vi "Read U64.vi"(8 "error in":errorcluster, 10 "register name":string, 11 "session in":u32) -> (0 "error out":errorcluster, 2 "value out":u64, 3 "session out":u32)   [LabVIEW 2018, in "Scalar IO Operations.lvlib"]
uses:
  Scalar IO Operations.lvlib
  NiFpga.dll
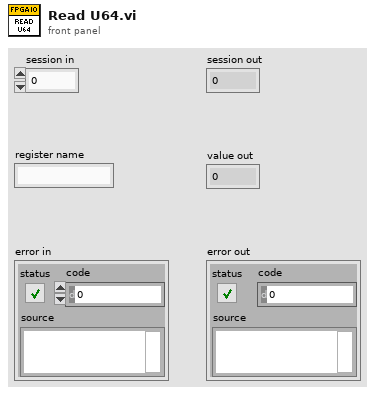
[diagram p1: front panel]
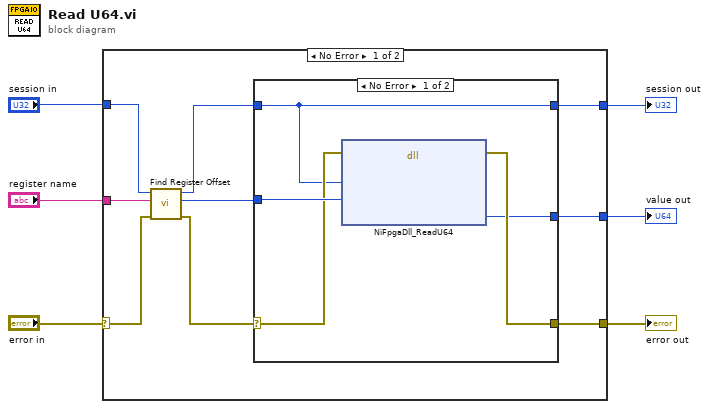
[diagram p0: block diagram]
diagram:
  n1 = case shown="No Error" "error in" {
    selector: "error in" -> [w7 w24]
    tunnel: [w15 w24] -> w6
    tunnel: [w14 _] -> w5
    tunnel: [w13 w23] -> w4
    tunnel: "session in" -> [w11 w23]
    tunnel: "register name" -> [w8 _]
    frame No Error {
      n2 = call "Find Register Offset.vi"("error in (no error)"=w7, "register name"=w8, "session in"=w11) -> ("error out"=w9:errorcluster, "resource offset"=w12:u32, "session out"=w10:u32)  [unwired: 6 in]
      n3 = case shown="No Error" w9 {
        selector: w9 -> [w17 w22]
        tunnel: w10 -> [w16 w21]
        tunnel: [w20 w22] -> w15
        tunnel: [w19 _] -> w14
        tunnel: w12 -> [w18 _]
        tunnel: [w16 w21] -> w13
        frame No Error {
          n4 = dll-call lib="NiFpga.*" fn="NiFpgaDll_ReadU64"(error in=w17, "session"=w16, "offset"=w18) -> (error out=w20:errorcluster, "value"=w19:u64)  [unwired: 6 in, 1 out]
        }
        frame Error {
        }
      }
    }
    frame Error {
    }
  }
  "error out" <- w6
  "session out" <- w4
  "value out" <- w5
